vi "Autonomous Play Execution.vi"(1 "Play 1":T1) -> (0 "All Robot Commands Out":T3)   [LabVIEW 2016]
uses:
  Subsystems/All Robot Commands.ctl
  Subsystems/Drive and Climb SS/Drive + Climb Commands 2017.ctl
  Subsystems/Gear Delivery SS/Gear Delivery Commands.ctl
  Subsystems/Conveyor and Shooter SS/Conveyor and Shooter Commands.ctl
  Subsystems/Ball Intake SS/Ball Intake Commands.ctl
  Autonomous Play Definition.ctl
  Autonomous Commands/Autonomous Command Names.ctl
  Global Variables/Autonomous Exec Info.vi
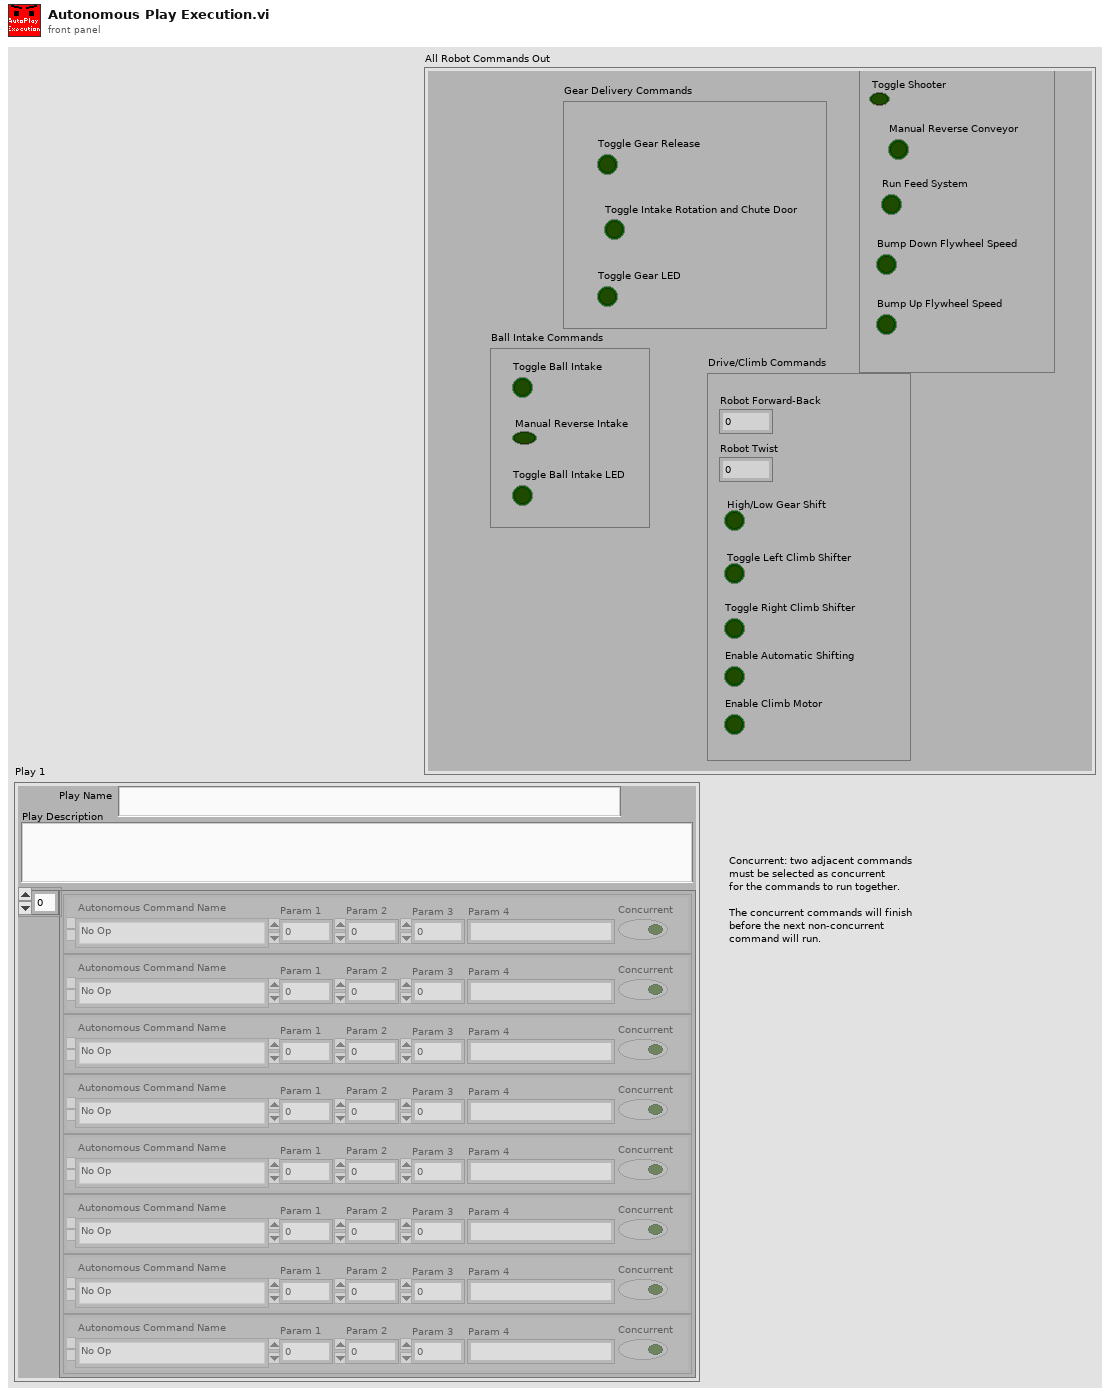
[diagram p1: front panel]
types:
  T1 = typedef "Autonomous Play Definition.ctl" = cluster{"Play Name":string, "Command List":cluster{"Param 1":dbl, "Param 2":dbl, "Autonomous Command Name":T2, "Concurrent":bool, "Param 3":dbl, "Param 4":string}[], "Play Description":string}
  T2 = typedef "Autonomous Command Names.ctl" = enum16{"No Op", "Command Drive+Climb Shift", "Command Wait", "Command Deliver Gear", "Command Buffer", "Command Drive Path", "Command Drive Time", "Command Shoot", "Command Turn to Heading", "Command Run Conveyor", "Command Spinup Shooter", "Command Deliver Gear Front", "Command Toggle Intake Rotation", "DO NOT USE", "Command Agitate Hopper", "Command Pre-Buffer", "Command Turn to Target", "Command Deliver Gear with Safety", "Command Drive Time with IMU", "Command Drive to Encoders"}
  T3 = typedef "All Robot Commands.ctl" = cluster{"Drive/Climb Commands":T4, "Gear Delivery Commands":T5, "Shooter and Conveyor Commands":T6, "Ball Intake Commands":T7}
  T4 = typedef "Drive + Climb Commands 2017.ctl" = cluster{"Robot Forward-Back":dbl, "Robot Twist":dbl, "High/Low Gear Shift":bool, "Toggle Left Climb Shifter":bool, "Toggle Right Climb Shifter":bool, "Enable Automatic Shifting":bool, "Enable Climb Motor ":bool}
  T5 = typedef "Gear Delivery Commands.ctl" = cluster{"Toggle Gear Release":bool, "Toggle Intake Rotation and Chute Door":bool, "Toggle Gear LED":bool}
  T6 = typedef "Conveyor and Shooter Commands.ctl" = cluster{"Toggle Shooter":bool, "Manual Reverse Conveyor":bool, "Run Feed System":bool, "Bump Down Flywheel Speed":bool, "Bump Up Flywheel Speed":bool}
  T7 = typedef "Ball Intake Commands.ctl" = cluster{"Toggle Ball Intake":bool, "Manual Reverse Intake":bool, "Toggle Ball Intake LED":bool}
  T8 = cluster{"Param 1":dbl, "Param 2":dbl, "Autonomous Command Name":T2, "Concurrent":bool, "Param 3":dbl, "Param 4":string}[]
  T9 = cluster{"Param 1":dbl, "Param 2":dbl, "Autonomous Command Name":T2, "Concurrent":bool, "Param 3":dbl, "Param 4":string}
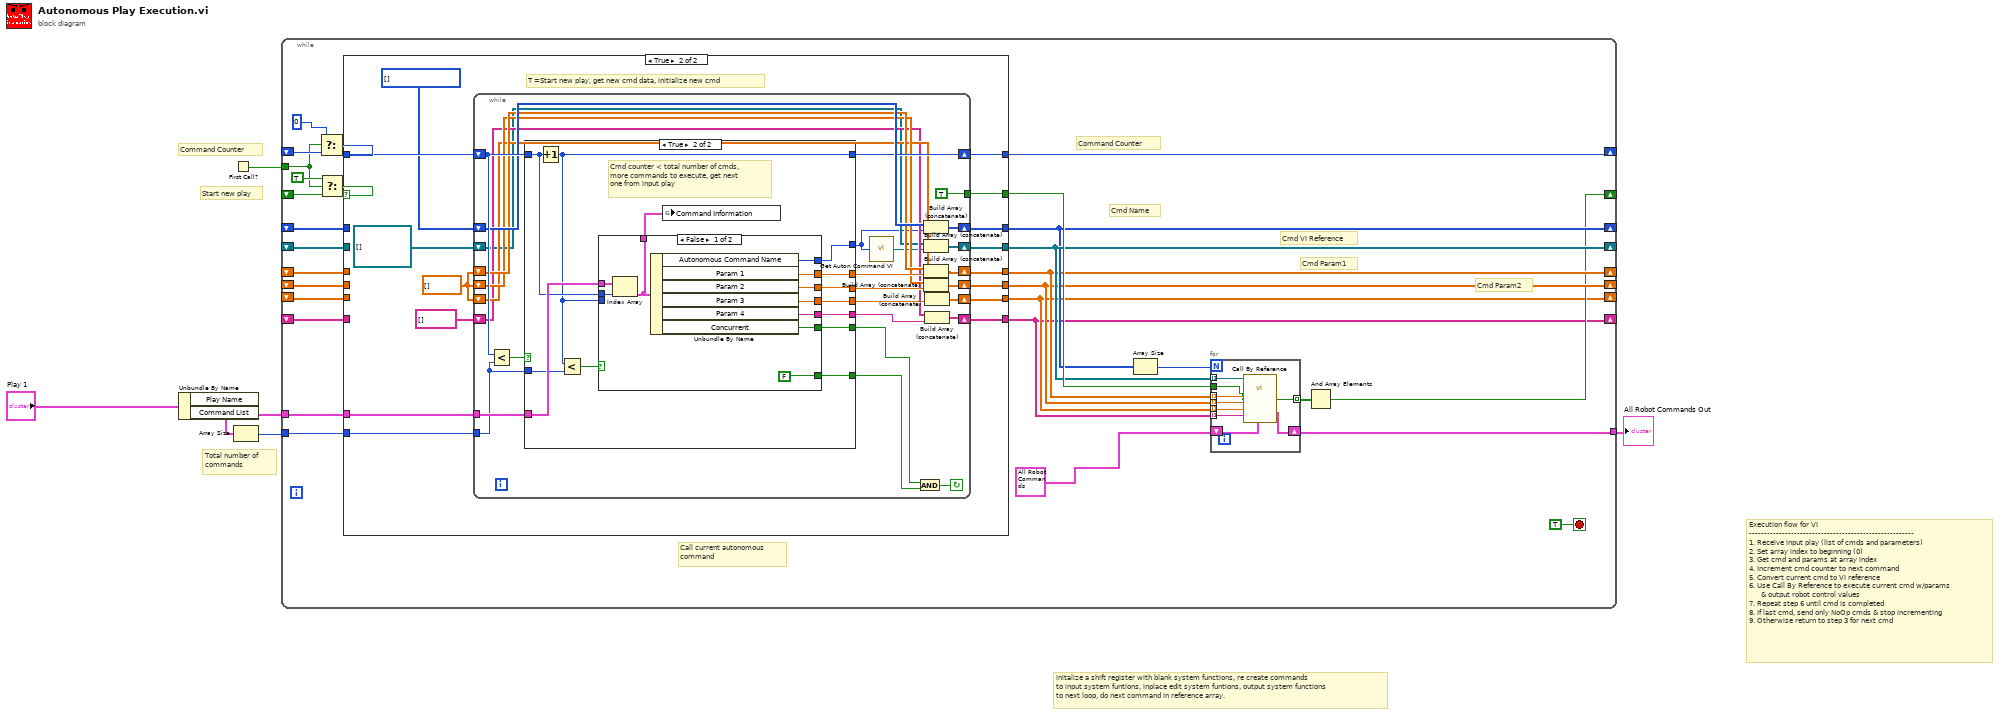
[diagram p0: block diagram]
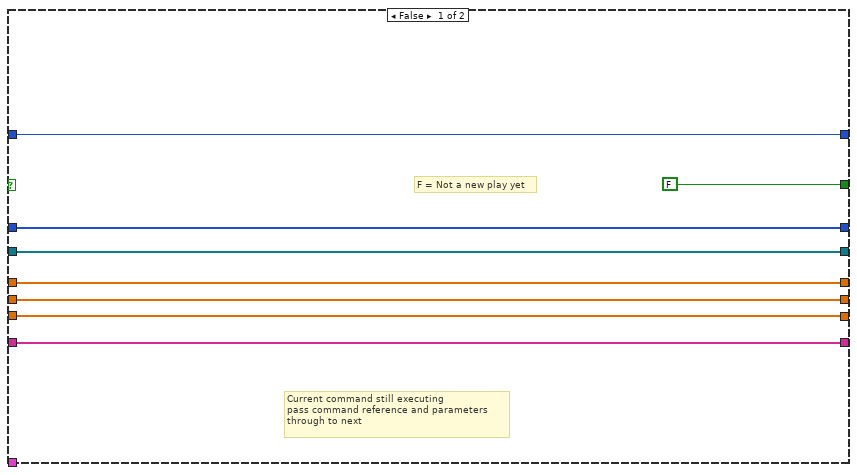
[diagram p2: hidden frame]
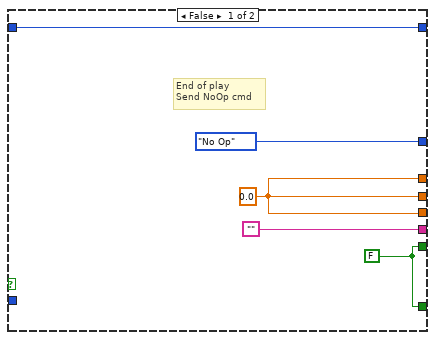
[diagram p3: hidden frame]
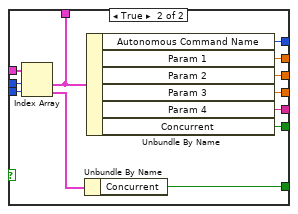
[diagram p4: hidden frame]
diagram:
  # "initalize a shift register with blank system functions, re create commands\nto input system funtions, inplace edit system funtions, output system functions\nto next loop, do next command in reference array."
  # "Execution flow for VI\n-------------------------------------------------------\n1. Receive input play (list of cmds and parameters)\n2. Set array index to beginning (0)\n3. Get cmd and params at array index\n4. Increment cmd counter to next command\n5. Convert current cmd to VI reference\n6. Use Call By Reference to execute current cmd w/params\n      & output robot control values\n7. Repeat step 6 until cmd is completed\n8. If last cmd, send only NoOp cmds & stop incrementing \n9. Otherwise return to step 3 for next cmd"
  # "Start new play"
  # "Total number of \ncommands"
  # "Command Counter"
  n1 = Unbundle By Name("Play 1") -> ("Command List"=w4:T8)  [unwired: 1 out]
  n2 = First Call?() -> (First Call?: T/F=w3:bool)
  n3 = Array Size(array=w4) -> (size(s)=w5:i32)
  n4 = while {
    tunnel: w4 -> [w32]
    tunnel: w5 -> [w29]
    shift-right: [w31] -> _
    shift-left: _ -> [w25]
    shift-right: [w13] -> _
    shift-left: _ -> [w23]
    shift-right: [w16] -> _
    shift-left: _ -> [w19]
    shift-right: [w33] -> _
    shift-left: _ -> [w14]
    shift-right: [w15] -> _
    shift-left: _ -> [w20]
    shift-right: [w18] -> _
    shift-left: _ -> [w28]
    tunnel: w3 -> [w21]
    tunnel: [w12] -> w2
    shift-right: [w11] -> _
    shift-left: _ -> [w10]
    shift-right: [w9] -> _
    shift-left: _ -> [w8]
    stop <- TRUE stop-if-true
    # "Cmd Name"
    # "Cmd Param2"
    # "Cmd Param1"
    # "Cmd VI Reference"
    # "Command Counter"
    # "Call current autonomous\ncommand"
    n5 = Select(t=0, s=w21, f=w25) -> (s? t:f=w26:i32)
    n6 = Select(t=TRUE, s=w21, f=w23) -> (s? t:f=w27:bool)
    n7 = case shown="True" w27 {
      tunnel: w32 -> [_ w66]
      tunnel: w26 -> [w51 w62]
      tunnel: [w49 w65] -> w15
      tunnel: [w48 w64] -> w16
      tunnel: [w51 w60] -> w31
      tunnel: [FALSE w63] -> w34
      tunnel: w29 -> [_ w61]
      tunnel: w28 -> [w47 _]
      tunnel: w20 -> [w49 _]
      tunnel: w19 -> [w48 _]
      tunnel: [w46 w54] -> w33
      tunnel: [w47 w59] -> w18
      tunnel: w14 -> [w46 _]
      tunnel: [w45 w53] -> w11
      tunnel: [w44 w52] -> w9
      tunnel: w10 -> [w45 _]
      tunnel: w8 -> [w44 _]
      frame False {
        # "F = Not a new play yet"
        # "Current command still executing\npass command reference and parameters \nthrough to next"
      }
      frame True {
        w58 = T2[] [] items=["No Op", "Command Drive+Climb Shift", "Command Wait", "Command Deliver Gear", "Command Buffer", "Command Drive Path", "Command Drive Time", "Command Shoot", "Command Turn to Heading", "Command Run Conveyor", "Command Spinup Shooter", "Command Deliver Gear Front", "Command Toggle Intake Rotation", "DO NOT USE", "Command Agitate Hopper", "Command Pre-Buffer", "Command Turn to Target", "Command Deliver Gear with Safety", "Command Drive Time with IMU", "Command Drive to Encoders"]
        w57 = dbl[] []
        # "T =Start new play, get new cmd data, initialize new cmd"
        n8 = while {
          tunnel: w66 -> [w91]
          tunnel: [TRUE] -> w63
          tunnel: w61 -> [w79]
          shift-right: [w88] -> w60
          shift-left: w62 -> [w93]
          shift-right: [w87] -> w64
          shift-left: w57 -> [w85]
          shift-right: [w84] -> w65
          shift-left: w57 -> [w83]
          shift-right: [w81] -> w59
          shift-left: w58 -> [w92]
          shift-right: [w75] -> w53
          shift-left: w57 -> [w76]
          shift-right: [w73] -> w52
          shift-left: string[] [] -> [w72]
          shift-right: [w70] -> w54
          shift-left: refnum<vi>[] [] -> [w69]
          stop <- w80 continue-if-true
          n9 = Less?(x=w93, y=w79) -> (x < y?=w89:bool)
          n10 = case shown="True" w89 {
            tunnel: w91 -> [_ w111]
            tunnel: [w94 w110] -> w82
            tunnel: [w94 w109] -> w86
            tunnel: w93 -> [w98 w108]
            tunnel: [w98 w103] -> w88
            tunnel: [Autonomous_Command_Names."No Op" ("Autonomous Command Name") w107] -> w67
            tunnel: w79 -> [_ w106]
            tunnel: [w96 w104] -> w78
            tunnel: [w96 w102] -> w77
            tunnel: [w94 w101] -> w74
            tunnel: ["" w100] -> w71
            frame False {
              w96 = FALSE ("Concurrent")
              w94 = 0.0 ("Param 2")
              # "End of play\nSend NoOp cmd"
            }
            frame True {
              # "Cmd counter < total number of cmds,\nmore commands to execute, get next\none from input play"
              n11 = Increment(x=w108) -> (x+1=w103:i32)
              n12 = Less?(x=w103, y=w106) -> (x < y?=w105:bool)
              n13 = case shown="False" w105 {
                tunnel: w111 -> [w116 w133]
                tunnel: [w120 w132] -> w110
                tunnel: [w119 w131] -> w109
                tunnel: w108 -> [w117 w130]
                tunnel: [w118 w129] -> w107
                tunnel: [FALSE ("Concurrent") w128] -> w104
                tunnel: w103 -> [_ w127]
                tunnel: [w115 w125] -> w102
                tunnel: [w114 w124] -> w101
                tunnel: [w113 w123] -> w100
                tunnel: [w112 w122] -> w99
                frame False {
                  n14 = Index Array(array=w116, index=w117) -> (element=w112:T9)
                  n15 = Unbundle By Name(w112) -> ("Autonomous Command Name"=w118:T2, "Param 1"=w119:dbl, "Param 2"=w120:dbl, "Param 3"=w114:dbl, "Param 4"=w113:string, "Concurrent"=w115:bool)
                }
                frame True {
                  n16 = Index Array(array=w133, index #1=w130, index #2=w127) -> (element #1=w122:T9, element #2=w126:T9)
                  n17 = Unbundle By Name(w126) -> ("Concurrent"=w128:bool)
                  n18 = Unbundle By Name(w122) -> ("Autonomous Command Name"=w129:T2, "Param 1"=w131:dbl, "Param 2"=w132:dbl, "Param 3"=w124:dbl, "Param 4"=w123:string, "Concurrent"=w125:bool)
                }
              }
              n19 = global write "Autonomous Exec Info.vi" "Command Information"(w99) -> ()
            }
          }
          n20 = call "Get Auton Command VI.vi"("Autonomous Command Name"=w67) -> ("VI Refnum"=w68:refnum<vi>)
          n21 = And(x=w77, y=w78) -> (x .and. y?=w80:bool)
          n22 = Build Array (concatenate)(w92, w67) -> (w81:T2[])
          n23 = Build Array (concatenate)(w69, w68) -> (w70:refnum<vi>[])
          n24 = Build Array (concatenate)(w85, w86) -> (w87:dbl[])
          n25 = Build Array (concatenate)(w83, w82) -> (w84:dbl[])
          n26 = Build Array (concatenate)(w76, w74) -> (w75:dbl[])
          n27 = Build Array (concatenate)(w72, w71) -> (w73:string[])
        }
      }
    }
    n28 = Array Size(array=w18) -> (size(s)=w17:i32)
    n29 = for {
      N: w17 -> [_]
      tunnel: w33 -> [w37] mode=indexing
      tunnel: w16 -> [w43] mode=indexing
      tunnel: w15 -> [w42] mode=indexing
      tunnel: w34 -> [w38]
      shift-right: [w35] -> w12
      shift-left: T3 {"Drive/Climb Commands"={"Robot Forward-Back"=0.0, "Robot Twist"=0.0, "High/Low Gear Shift"=FALSE, "Toggle Left Climb Shifter"=FALSE, "Toggle Right Climb Shifter"=FALSE, "Enable Automatic Shifting"=FALSE, "Enable Climb Motor "=FALSE}, "Gear Delivery Commands"={"Toggle Gear Release"=FALSE, "Toggle Intake Rotation and Chute Door"=FALSE, "Toggle Gear LED"=FALSE}, "Shooter and Conveyor Commands"={"Toggle Shooter"=FALSE, "Manual Reverse Conveyor"=FALSE, "Run Feed System"=FALSE, "Bump Down Flywheel Speed"=FALSE, "Bump Up Flywheel Speed"=FALSE}, "Ball Intake Commands"={"Toggle Ball Intake"=FALSE, "Manual Reverse Intake"=FALSE, "Toggle Ball Intake LED"=FALSE}} ("All Robot Commands") -> [w36]
      tunnel: w11 -> [w41] mode=indexing
      tunnel: w9 -> [w40] mode=indexing
      tunnel: [w39] -> w6 mode=indexing
      n30 = call-by-ref "?"(reference=w37, "Robot System Functions In"=w36, "Startup"=w38, "String Parameter"=w40, "Cmd Parameter 3"=w41, "Cmd Parameter 2"=w42, "Cmd Parameter 1"=w43) -> ("Robot System Functions Out"=w35:T3, "Completed"=w39:bool)  [unwired: 1 in, 2 out]
    }
    n31 = And Array Elements(Boolean array=w6) -> (logical AND=w13:bool)
  }
  "All Robot Commands Out" <- w2
